vi "Read Mapping Mode.vi"(9 "Scale in":refnum<class "Scale.lvclass">) -> (3 "Scale out":refnum<class "Scale.lvclass">, 4 "Mapping Mode":u8)   [LabVIEW 2014, in "Scale.lvclass"]
uses:
  Scale.lvclass
  Scale.lvclass/Scale.ctl
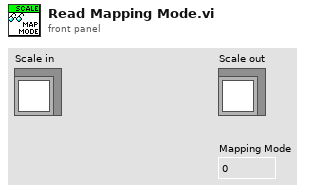
[diagram p1: front panel]
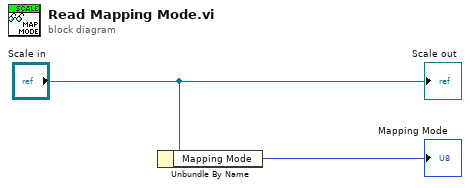
[diagram p0: block diagram]
diagram:
  n1 = Unbundle By Name("Scale in") -> ("Mapping Mode"=→"Mapping Mode":u8)
  "Scale out" <- "Scale in"
